vi "Map_InitMap.vi"(10 "Map Objects In":T1, 11 "Game State In":T4) -> (2 "Map Objects Out":T1, 3 "Game State Out":T4)   [LabVIEW 2020]
uses:
  Controls/Game_State.ctl
  Controls/Player_LocationInfo.ctl
  Controls/Player_LocationInfoAxis.ctl
  Controls/Map_Position.ctl
  Controls/Map_Objects.ctl
  Controls/Map_Object.ctl
  Map_GetMaps.vi
  <vilib>/Utility/file.llb/Application Directory.vi
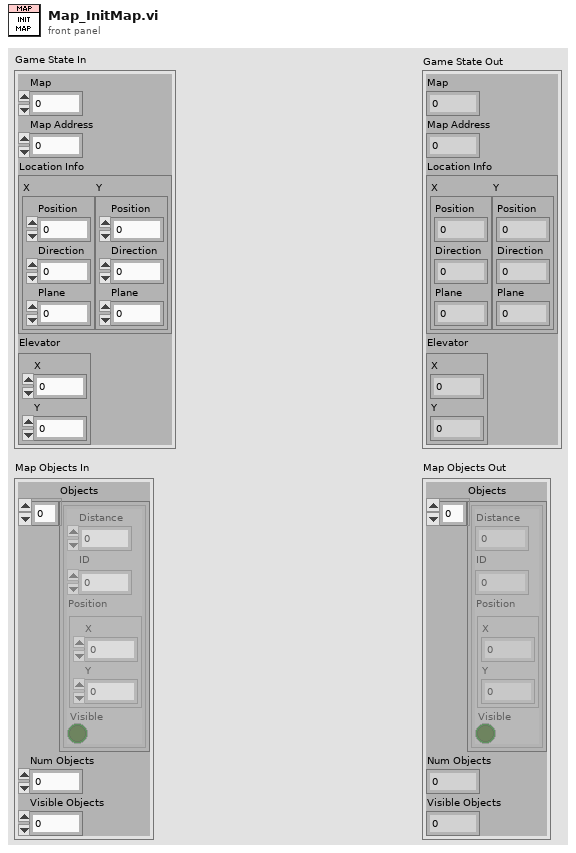
[diagram p1: front panel]
types:
  T1 = typedef "Map_Objects.ctl" = cluster{"Objects":T2[], "Num Objects":i16, "Visible Objects":i16}
  T2 = typedef "Map_Object.ctl" = cluster{"Distance":fxp<+/-,32,16>, "ID":u8, "Position":T3, "Visible":bool}
  T3 = typedef "Map_Position.ctl" = cluster{"X":fxp<+/-,32,16>, "Y":fxp<+/-,32,16>}
  T4 = typedef "Game_State.ctl" = cluster{"Map":u8, "Map Address":u32, "Location Info":T5, "Elevator":T3}
  T5 = typedef "Player_LocationInfo.ctl" = cluster{"X":T6, "Y":T6}
  T6 = typedef "Player_LocationInfoAxis.ctl" = cluster{"Position":fxp<+/-,32,16>, "Direction":fxp<+/-,32,16>, "Plane":fxp<+/-,32,16>}
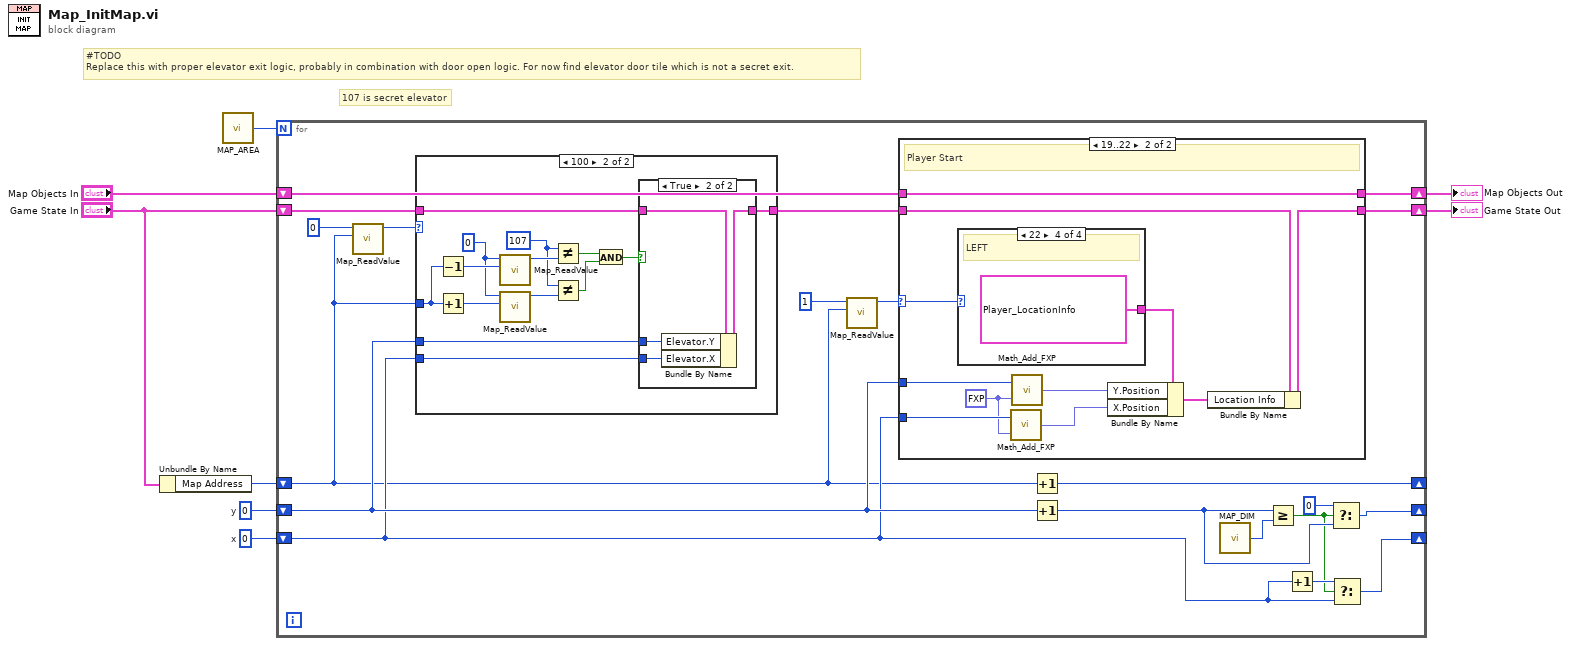
[diagram p0: block diagram]
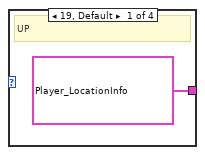
[diagram p3: hidden frame]
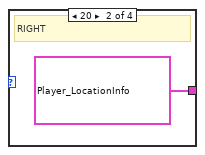
[diagram p4: hidden frame]
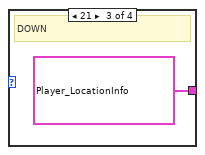
[diagram p5: hidden frame]
diagram:
  w7 = i16 0  # y
  w8 = i16 0  # x
  # "#TODO\nReplace this with proper elevator exit logic, probably in combination with door open logic. For now find elevator door tile which is not a secret exit."
  # "107 is secret elevator"
  n1 = Unbundle By Name("Game State In") -> ("Map Address"=w6:u32)
  n2 = call "MAP_AREA.vi"() -> ("MAP_DIM"=w4:i16)
  n3 = for {
    N: w4 -> [_]
    shift-right: [w21] -> _
    shift-left: w6 -> [w11]
    shift-right: [w18] -> _
    shift-left: w8 -> [w12]
    shift-right: [w19] -> _
    shift-left: w7 -> [w13]
    shift-right: [w20] -> w3
    shift-left: "Game State In" -> [w15]
    shift-right: [w9] -> w1
    shift-left: "Map Objects In" -> [w10]
    n4 = call "Map_ReadValue.vi"("Address"=w11, "Plane"=u8 0) -> ("Value"=w16:u8)  [unwired: 9 in]
    n5 = case shown="100" w16 {
      tunnel: w15 -> [w46 w59]
      tunnel: [w46 w60] -> w14
      tunnel: w13 -> [_ w58]
      tunnel: w12 -> [_ w57]
      tunnel: w11 -> [_ w55]
      frame Default {
      }
      frame 100 {
        w47 = u8 0 ("Plane")
        w52 = u8 107 ("x")
        n6 = Decrement(x=w55) -> (x-1=w54:u32)
        n7 = Increment(x=w55) -> (x+1=w56:u32)
        n8 = call "Map_ReadValue.vi"("Address"=w54, "Plane"=w47) -> ("Value"=w53:u8)  [unwired: 9 in]
        n9 = call "Map_ReadValue.vi"("Address"=w56, "Plane"=w47) -> ("Value"=w51:u8)  [unwired: 9 in]
        n10 = Not Equal?(x=w52, y=w53) -> (x != y?=w50:bool)
        n11 = Not Equal?(x=w52, y=w51) -> (x != y?=w49:bool)
        n12 = And(x=w50, y=w49) -> (x .and. y?=w48:bool)
        n13 = case shown="True" w48 {
          tunnel: [w61 w65] -> w60
          tunnel: w59 -> [w61 w64]
          tunnel: w58 -> [_ w63]
          tunnel: w57 -> [_ w62]
          frame False {
          }
          frame True {
            n14 = Bundle By Name(cluster=w64, "Elevator.Y"=w63, "Elevator.X"=w62) -> (w65:T4)
          }
        }
      }
    }
    n15 = call "Map_ReadValue.vi"("Address"=w11, "Plane"=u8 1) -> ("Value"=w22:u8)  [unwired: 9 in]
    n16 = case shown="19..22" w22 {
      selector: w22 -> [_ w36]
      tunnel: w14 -> [w30 w34]
      tunnel: [w30 w33] -> w20
      tunnel: w13 -> [_ w41]
      tunnel: w12 -> [_ w39]
      tunnel: w10 -> [w29 w31]
      tunnel: [w29 w31] -> w9
      frame Default {
      }
      frame 19..22 {
        w37 = fxp<+/-,32,16> 0.5 ("y")
        # "Player Start"
        n17 = case shown="22" w36 {
          tunnel: [T5 {"X"={"Position"=0.0, "Direction"=-1.0, "Plane"=0.0}, "Y"={"Position"=0.0, "Direction"=0.0, "Plane"=0.660003662109375}} T5 {"X"={"Position"=0.0, "Direction"=0.0, "Plane"=0.660003662109375}, "Y"={"Position"=0.0, "Direction"=1.0, "Plane"=0.0}} T5 {"X"={"Position"=0.0, "Direction"=1.0, "Plane"=0.0}, "Y"={"Position"=0.0, "Direction"=0.0, "Plane"=-0.660003662109375}} T5 {"X"={"Position"=0.0, "Direction"=0.0, "Plane"=-0.660003662109375}, "Y"={"Position"=0.0, "Direction"=-1.0, "Plane"=0.0}}] -> w35
          frame 19, Default {
            # "UP"
          }
          frame 20 {
            # "RIGHT"
          }
          frame 21 {
            # "DOWN"
          }
          frame 22 {
            # "LEFT"
          }
        }
        n18 = call "Math_Add_FXP.vi"("y"=w37, "x"=w39) -> ("x*y"=w38:fxp<+/-,32,16>)
        n19 = call "Math_Add_FXP.vi"("y"=w37, "x"=w41) -> ("x*y"=w40:fxp<+/-,32,16>)
        n20 = Bundle By Name(cluster=w35, "Y.Position"=w40, "X.Position"=w38) -> (w32:T5)
        n21 = Bundle By Name(cluster=w34, "Location Info"=w32) -> (w33:T4)
      }
    }
    n22 = Increment(x=w11) -> (x+1=w21:u32)
    n23 = Increment(x=w13) -> (x+1=w26:i16)
    n24 = call "MAP_DIM.vi"() -> ("MAP_DIM"=w27:i16)
    n25 = Greater Or Equal?(x=w26, y=w27) -> (x >= y?=w23:bool)
    n26 = Increment(x=w12) -> (x+1=w24:i16)
    n27 = Select(t=i16 0, s=w23, f=w26) -> (s? t:f=w19:i16)
    n28 = Select(t=w24, s=w23, f=w12) -> (s? t:f=w18:i16)
  }
  "Game State Out" <- w3
  "Map Objects Out" <- w1
